vi "whiletercero.vi"() -> ()   [LabVIEW 2012]
panel:
  out "x":dbl
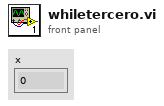
[diagram p1: front panel]
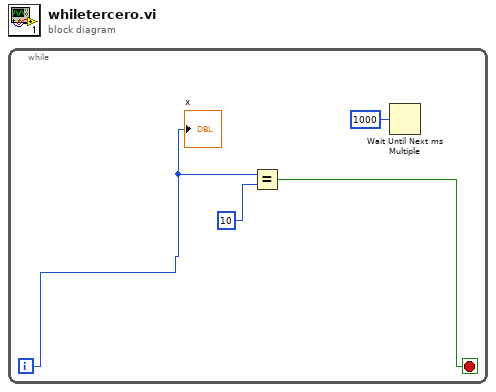
[diagram p0: block diagram]
diagram:
  n1 = while {
    i -> [w3]
    stop <- w1 stop-if-true
    n2 = Equal?(x=w3, y=10 ("x")) -> (x = y?=w1:bool)
    n3 = Wait Until Next ms Multiple(millisecond multiple=u32 1000) -> ()  [unwired: 1 out]
    "x" <- w3
  }
